vi "GET BEAD PROFILE ORNL Ver1.vi"() -> ()   [LabVIEW 2016]
uses:
  <vilib>/Platform/TimedLoop/XDataNode/timing_clust.ctl
  <vilib>/Platform/TimedLoop/XDataNode/nitl_modes.ctl
  <vilib>/Platform/TimedLoop/XDataNode/wakeup.ctl
  <vilib>/DAQmx/read.llb/DAQmx Read (Digital 1D Bool 1Chan 1Samp).vi
  <vilib>/DAQmx/write.llb/DAQmx Write (Digital Bool 1Line 1Point).vi
  <vilib>/DAQmx/read.llb/DAQmx Read (Analog DBL 1Chan 1Samp).vi
  <vilib>/DAQmx/miscellaneous.llb/DAQmx Fill In Error Info.vi
  <vilib>/Utility/file.llb/Write Delimited Spreadsheet (DBL).vi
  <vilib>/platform/TimedLoop/XDataNode/XDataNode.xnode
  <vilib>/Platform/TimedLoop/XDataNode/XDNodeRunTimeDep.lvlib
panel:
  in  "BIAS":dbl=-17.4
  out "Kuka Code":u32=31
  out "Print/Scan":bool
  in  "mm/Volt":dbl=6.0
  in  "Write To File?":bool
  out "Ready to Scan":bool
  in  "Keyence On/Open":bool
  out "Waveform Graph":waveform(dbl)(graph)={"t0"=timestamp(0 s since 1904-01-01), "dt"=0.125, "Y"=array[4552 elements]}
  in  "Robot Speed":dbl=25.0
  out "Position":dbl=568.875
  out "Height":dbl=-17.417521476745605 format="%0.2f"
  out "ScanTrigger":bool
  in  "stop":bool
  # "MODE"
  # "mm/s"
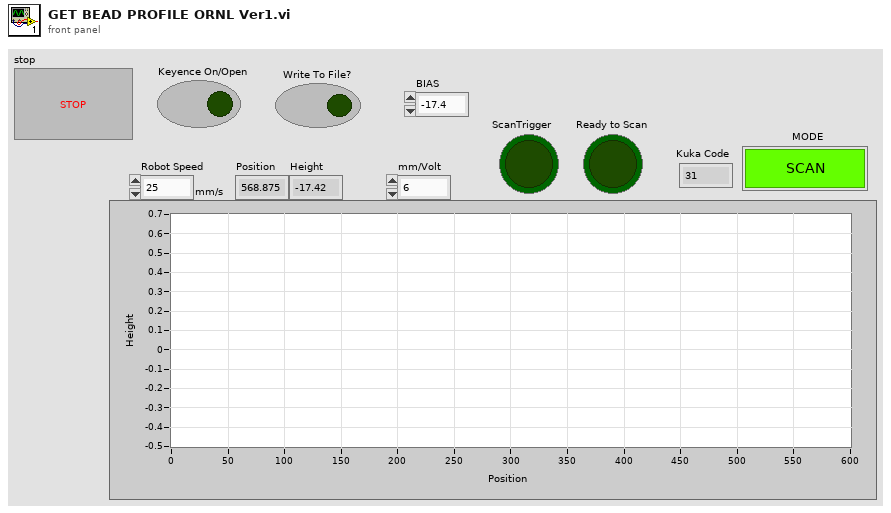
[diagram p1: front panel]
types:
  T1 = typedef "XDNodeRunTimeDep.lvlib/timing_clust.ctl" = cluster{"Expected End [f-1]":u64, "Actual End [f-1]":u64, "Finished Late? [f-1]":bool, "Expected End [i-1]":u64, "Actual End [i-1]":u64, "Finished Late? [i-1]":bool, "Expected Start [i]":u64, "Actual Start [i]":u64, "Expected Start [f]":u64, "Actual Start [f]":u64, "Source Name":string, "Structure Name":string, "Period":i64, "Deadline":i64, "Offset":i64, "Start":i64, "Priority":i32, "Timeout":i32, "Mode":T2, "Wakeup Reason":T3, "Error":errorcluster, "Source Type":string, "Secondary Source Type":string, "Global End Time":u64, "Global Start Time":u64, "Frame Duration":u64, "Iteration Duration":u64, "Assigned CPU":i32, "I/O Scan Engine Mode":u32}
  T2 = typedef "XDNodeRunTimeDep.lvlib/nitl_modes.ctl" = enum32{"No Change", "Process missed periods, maintain original phase", "Discard missed periods, maintain original phase", "Process missed periods, ignore original phase", "Discard missed periods, ignore original phase"}
  T3 = typedef "XDNodeRunTimeDep.lvlib/wakeup.ctl" = enum32{"Normal", "Aborted", "Asynchronous wakeup", "Timing source error", "Timed loop error", "Timeout"}
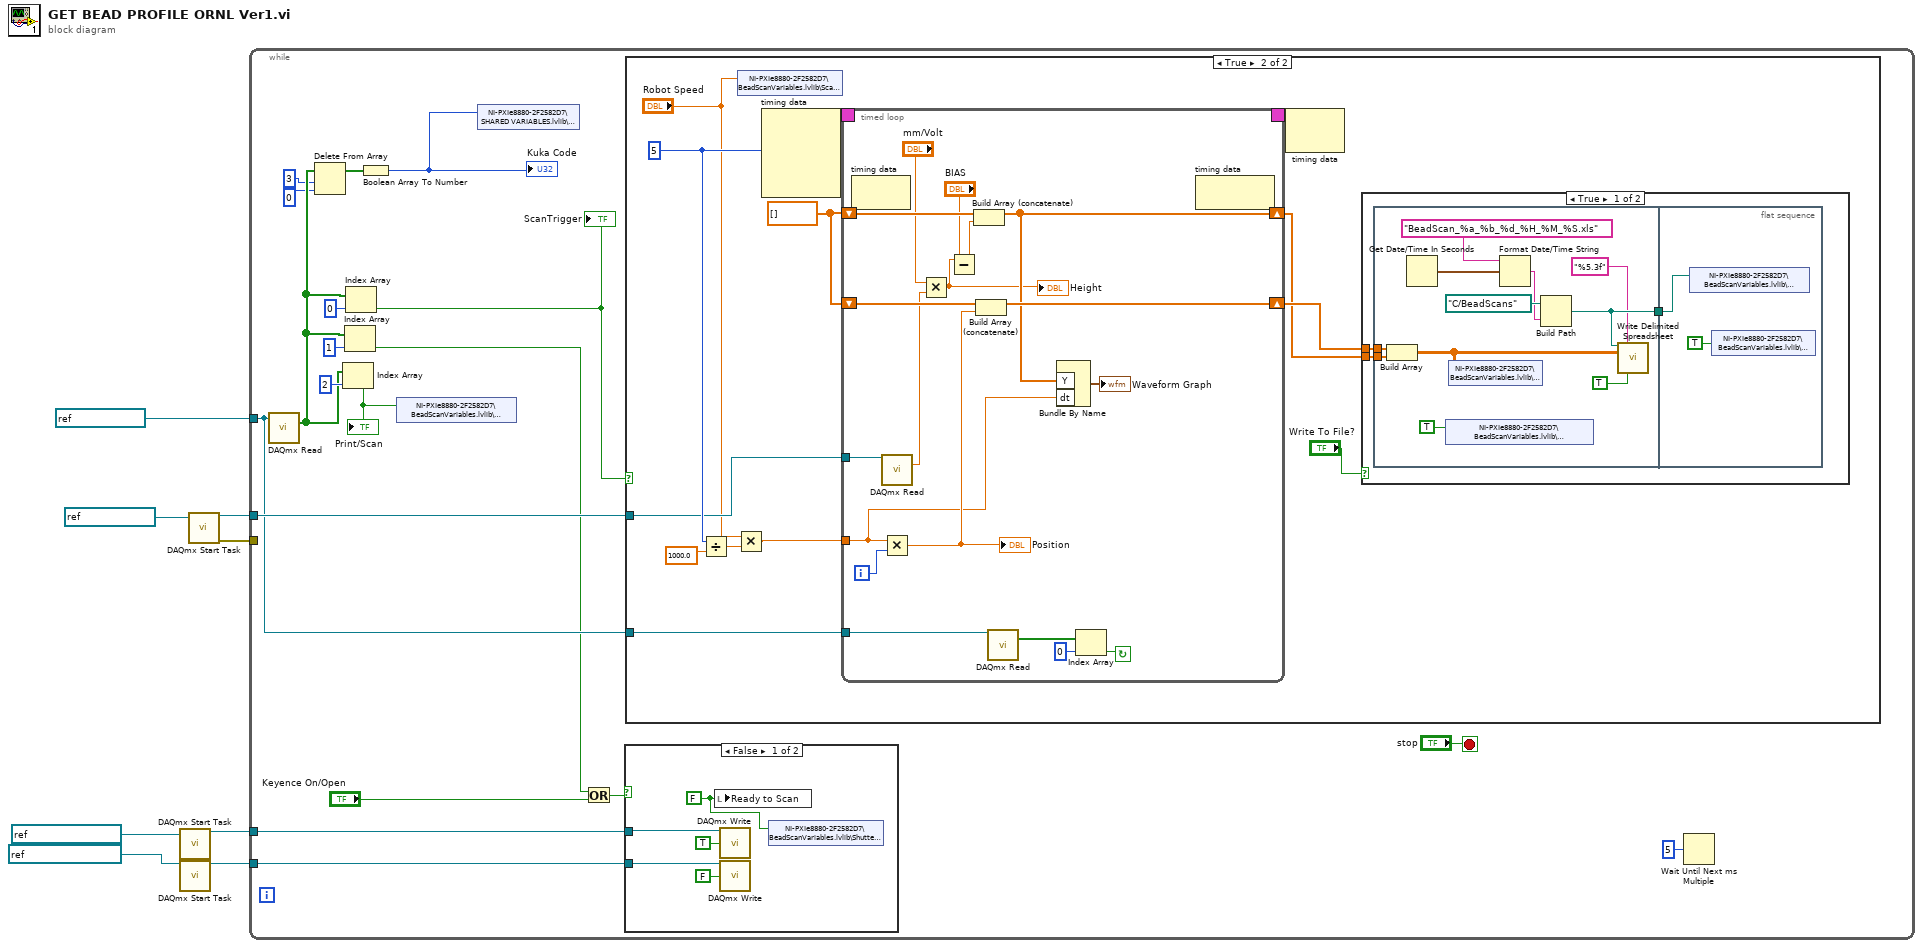
[diagram p0: block diagram]
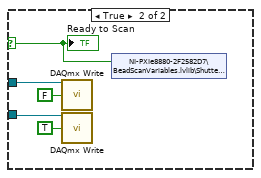
[diagram p2: hidden frame]
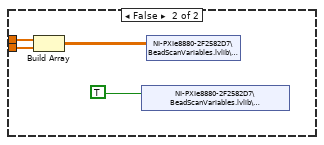
[diagram p4: hidden frame]
diagram:
  n1 = call <vilib>:"DAQmx Start Task.vi"("task/channels in"=refnum<k21> "Keyence Enable" ("DAQmx Task Name")) -> ("task out"=w2:refnum<k21>, "error out"=w6:errorcluster)  [unwired: 13 in]
  n2 = call <vilib>:"DAQmx Start Task.vi"("task/channels in"=refnum<k21> "Keyence Shutter" ("DAQmx Task Name"), "error in"=w6) -> ("task out"=w3:refnum<k21>)  [unwired: 12 in, 1 out]
  n3 = call <vilib>:"DAQmx Start Task.vi"("task/channels in"=refnum<k21> "Keyence BH" ("DAQmx Task Name")) -> ("task out"=w8:refnum<k21>, "error out"=w7:errorcluster)  [unwired: 13 in]
  n4 = while {
    tunnel: w8 -> [w26]
    tunnel: w7 -> [_]
    tunnel: w3 -> [w22]
    tunnel: w2 -> [w23]
    tunnel: refnum<k21> "Kuka Inputs" ("DAQmx Task Name") -> [w19]
    stop <- "stop" stop-if-true
    n5 = call-poly <vilib>:"DAQmx Read.vi"("task/channels in"=w19) -> ("data"=w15:bool[])  [unwired: 12 in, 2 out]
    n6 = Delete From Array(array=w15, length=3, index=0) -> (array with subset deleted=w12:bool[])  [unwired: 1 out]
    n7 = Index Array(array=w15, index=2) -> (element=w11:bool)
    "Print/Scan" <- w11
    n8 = Index Array(array=w15, index=1) -> (element=w17:bool)
    n9 = Index Array(array=w15, index=0) -> (element=w20:bool)
    "ScanTrigger" <- w20
    n10 = Boolean Array To Number(Boolean array=w12) -> (number=w10:u32)
    "Kuka Code" <- w10
    n11 = shared-variable "NI-PXIe8880-2F2582D7\\BeadScanVariables.lvlib\\PRINTorSCAN"(w11) -> ()  [unwired: 1 in, 1 out]
    n12 = shared-variable "NI-PXIe8880-2F2582D7\\SHARED VARIABLES.lvlib\\Kuka Code"(w10) -> ()  [unwired: 1 in, 1 out]
    n13 = Or(x=w17, y="Keyence On/Open") -> (x .or. y?=w25:bool)
    n14 = case shown="False" w25 {
      selector: w25 -> [_ w34]
      tunnel: w23 -> [w31 w38]
      tunnel: w22 -> [w30 w37]
      frame False {
        w29 = FALSE
        n15 = local write "Ready to Scan"(w29) -> ()
        n16 = call-poly <vilib>:"DAQmx Write.vi"("task/channels in"=w31, "data"=TRUE) -> ()  [unwired: 11 in, 3 out]
        n17 = call-poly <vilib>:"DAQmx Write.vi"("task/channels in"=w30, "data"=FALSE) -> ()  [unwired: 11 in, 3 out]
        n18 = shared-variable "NI-PXIe8880-2F2582D7\\BeadScanVariables.lvlib\\Shutter Open"(w29) -> ()  [unwired: 1 in, 1 out]
      }
      frame True {
        n19 = call-poly <vilib>:"DAQmx Write.vi"("task/channels in"=w38, "data"=FALSE) -> ()  [unwired: 11 in, 3 out]
        n20 = call-poly <vilib>:"DAQmx Write.vi"("task/channels in"=w37, "data"=TRUE) -> ()  [unwired: 11 in, 3 out]
        n21 = shared-variable "NI-PXIe8880-2F2582D7\\BeadScanVariables.lvlib\\Shutter Open"(w34) -> ()  [unwired: 1 in, 1 out]
        "Ready to Scan" <- w34
      }
    }
    n22 = case shown="True" w20 {
      tunnel: w26 -> [_ w45]
      tunnel: w19 -> [_ w40]
      frame False {
      }
      frame True {
        w44 = dbl[] [] ("appended array")
        w47 = i64 5 ("Period")
        n23 = Divide(x=w47, y=1000.0) -> (x/y=w49:dbl)
        n24 = Multiply(x="Robot Speed", y=w49) -> (x*y=w46:dbl)
        n25 = shared-variable "NI-PXIe8880-2F2582D7\\BeadScanVariables.lvlib\\Scan Speed"("Robot Speed") -> ()  [unwired: 1 in, 1 out]
        n26 = node-c288(w47) -> (w51:T1)  [unwired: 3 in]
        n27 = timed-loop {
          timing: w51 -> [_]
          timing-out: [_] -> w50
          tunnel: w46 -> [w79]
          tunnel: w45 -> [w88]
          shift-right: [w80] -> w42
          shift-left: w44 -> [w84]
          shift-right: [w81] -> w43
          shift-left: w44 -> [w82]
          tunnel: w40 -> [w75]
          i -> [w89]
          stop <- w85 continue-if-true
          n28 = node-c288() -> ()  [unwired: 1 in, 1 out]
          n29 = call-poly <vilib>:"DAQmx Read.vi"("task/channels in"=w88) -> ("data"=w77:dbl)  [unwired: 12 in, 2 out]
          n30 = Multiply(x=w79, y=w89) -> (x*y=w83:dbl)
          "Position" <- w83
          n31 = Multiply(x="mm/Volt", y=w77) -> (x*y=w73:dbl)
          "Height" <- w73
          n32 = Subtract(x=w73, y="BIAS") -> (x-y=w74:dbl)
          n33 = Build Array (concatenate)(w84, w74) -> (w80:dbl[])
          n34 = Build Array (concatenate)(w82, w83) -> (w81:dbl[])
          n35 = call-poly <vilib>:"DAQmx Read.vi"("task/channels in"=w75) -> ("data"=w86:bool[])  [unwired: 12 in, 2 out]
          n36 = Bundle By Name("Y"=w80, "dt"=w79) -> (→"Waveform Graph":waveform(dbl))  [unwired: 1 in]
          n37 = Index Array(array=w86, index=0) -> (element=w85:bool)
          n38 = node-c288() -> ()  [unwired: 1 in, 1 out]
        }
        n39 = node-c288(w50) -> ()  [unwired: 1 out]
        n40 = case shown="True" "Write To File?" {
          tunnel: w43 -> [w54 w71]
          tunnel: w42 -> [w53 w70]
          frame True {
            n41 = flat-sequence {
              tunnel: w54 -> [w57]
              tunnel: w53 -> [w56]
              tunnel: [w61] -> w52
              tunnel: w52 -> [w67]
              frame #0 {
                n42 = Build Array(w57, w56) -> (w60:dbl[][])
                n43 = Get Date/Time In Seconds() -> (seconds since 1Jan1904=w64:timestamp)
                n44 = shared-variable "NI-PXIe8880-2F2582D7\\BeadScanVariables.lvlib\\BeadScanComplete"(TRUE ("transpose? (no:F)")) -> ()  [unwired: 1 in, 1 out]
                n45 = shared-variable "NI-PXIe8880-2F2582D7\\BeadScanVariables.lvlib\\ScanData"(w60) -> ()  [unwired: 1 in, 1 out]
                n46 = Format Date/Time String(time format string (%c)="BeadScan_%a_%b_%d_%H_%M_%S.xls", seconds (now)=w64) -> (date/time string=w62:string)  [unwired: 1 in]
                n47 = Build Path(base path=path "C:/BeadScans", name or relative path=w62) -> (appended path=w61:path)
                n48 = call-poly <vilib>:"Write Delimited Spreadsheet.vi"("file path (dialog if empty)"=w61, "format (%.3f)"="%5.3f", "2D data"=w60, "transpose? (no:F)"=TRUE) -> ()  [unwired: 10 in, 2 out]
              }
              frame #1 {
                n49 = shared-variable "NI-PXIe8880-2F2582D7\\BeadScanVariables.lvlib\\BeadScanPath"(w67) -> ()  [unwired: 1 in, 1 out]
                n50 = shared-variable "NI-PXIe8880-2F2582D7\\BeadScanVariables.lvlib\\FileWaiting"(TRUE) -> ()  [unwired: 1 in, 1 out]
              }
            }
          }
          frame False {
            n51 = Build Array(w71, w70) -> (w69:dbl[][])
            n52 = shared-variable "NI-PXIe8880-2F2582D7\\BeadScanVariables.lvlib\\BeadScanComplete"(TRUE) -> ()  [unwired: 1 in, 1 out]
            n53 = shared-variable "NI-PXIe8880-2F2582D7\\BeadScanVariables.lvlib\\ScanData"(w69) -> ()  [unwired: 1 in, 1 out]
          }
        }
      }
    }
    n54 = Wait Until Next ms Multiple(millisecond multiple=u32 5) -> ()  [unwired: 1 out]
  }
